vi "APS relative move.vi"(8 "error in (no error)":errorcluster caption="错误输入（无错误）", 9 "Max_Speed":i32, 10 "Distance":i32, 11 "Axis_ID":i32) -> (0 "error out":errorcluster caption="错误输出", 3 "function return":i32)   [LabVIEW 2017]
doc: "I32 FNTYPE APS_relative_move( I32 Axis_ID, I32 Distance, I32 Max_Speed );"
uses:
  APS168.dll
  APS168.lvlib
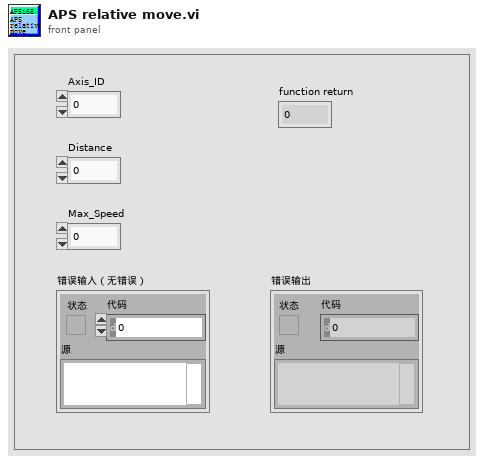
[diagram p1: front panel]
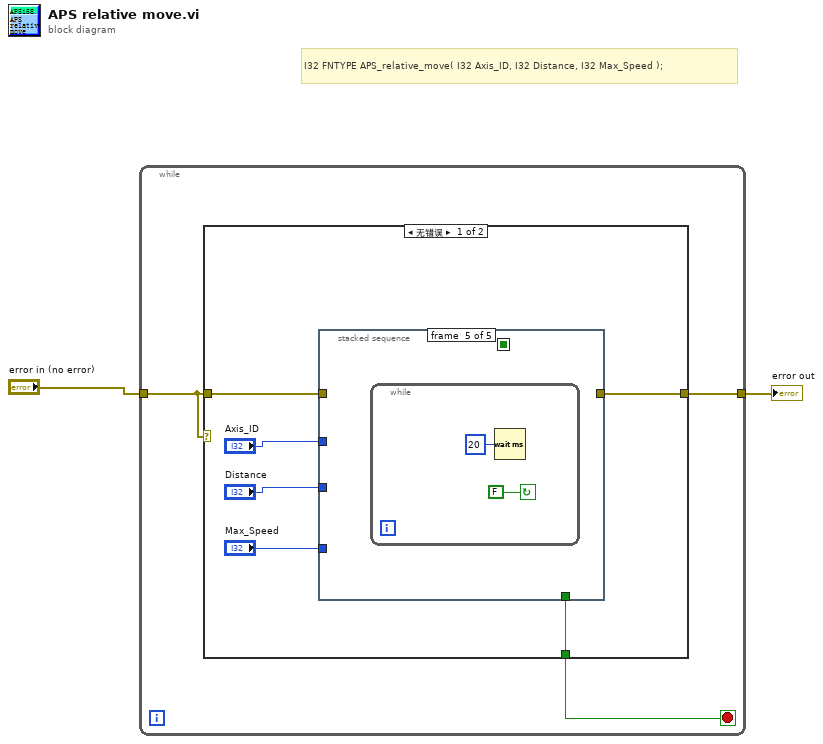
[diagram p0: block diagram]
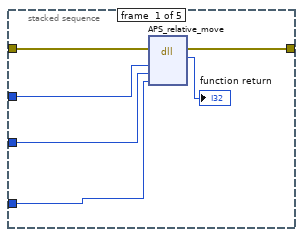
[diagram p2: hidden frame]
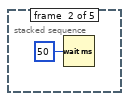
[diagram p3: hidden frame]
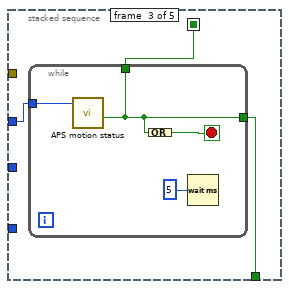
[diagram p4: hidden frame]
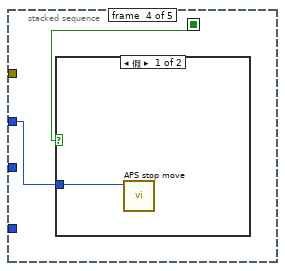
[diagram p5: hidden frame]
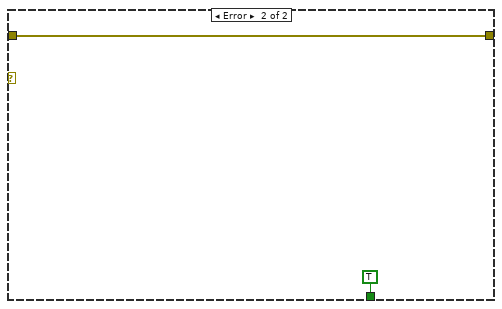
[diagram p7: hidden frame]
diagram:
  # "I32 FNTYPE APS_relative_move( I32 Axis_ID, I32 Distance, I32 Max_Speed );"
  n1 = while {
    tunnel: [w5] -> w2
    tunnel: "error in (no error)" -> [w4]
    stop <- w3 stop-if-true
    n2 = case shown="无错误" w4 {
      tunnel: [w11 w32] -> w5
      tunnel: w4 -> [w10 w32]
      tunnel: [w6 TRUE ("x与y?")] -> w3
      frame No Error {
        n3 = stacked-sequence {
          seq-local: [_ _ w20 _ _] -> [_ _ _ w27 _]
          tunnel: [_ _ w21 _ _] -> w6
          tunnel: w10 -> [w16 _ _ _ _]
          tunnel: [w15 _ _ _ _] -> w11
          tunnel: "Axis_ID" -> [w14 _ w19 w26 _]
          tunnel: "Distance" -> [w13 _ _ _ _]
          tunnel: "Max_Speed" -> [w12 _ _ _ _]
          frame #0 {
            n4 = dll-call lib="PTH2Labs E迈治LV范例testSubVIsADLINKLLB运动204cAPS168.*" fn="APS_relative_move"(error in=w16, "Axis_ID"=w14, "Distance"=w13, "Max_Speed"=w12) -> (error out=w15:errorcluster, →"function return":i32)  [unwired: 5 in, 1 out]
          }
          frame #1 {
            n5 = Wait (ms)(milliseconds to wait=u32 50 ("等待时间（毫秒）")) -> ()  [unwired: 1 out]
          }
          frame #2 {
            n6 = while {
              tunnel: w19 -> [w24]
              tunnel: [w22] -> w21
              tunnel: [w22] -> w20
              stop <- w23 stop-if-true
              n7 = call "APS motion status.vi"("Axis_ID"=w24) -> ("x与y?"=w22:bool)  [unwired: 9 in, 1 out]
              n8 = Compound Arithmetic op=OR(w22) -> (w23:bool)
              n9 = Wait (ms)(milliseconds to wait=u32 5 ("等待时间（毫秒）")) -> ()  [unwired: 1 out]
            }
          }
          frame #3 {
            n10 = case shown="假" w27 {
              tunnel: w26 -> [w28 _]
              frame False {
                n11 = call "APS stop move.vi"("Axis_ID"=w28) -> ()  [unwired: 9 in, 2 out]
              }
              frame True {
              }
            }
          }
          frame #4 {
            n12 = while {
              stop <- FALSE continue-if-true
              n13 = Wait (ms)(milliseconds to wait=u32 20 ("等待时间（毫秒）")) -> ()  [unwired: 1 out]
            }
          }
        }
      }
      frame Error {
      }
    }
  }
  "error out" <- w2
